vi "Create Arbitrary Waveform.vi"(4 "Arbitrary Waveform Data":dbl[](array[numeric]), 6 "Arbitrary Waveform Name (ARB1)":string="ARB1", 8 "error in (no error)":errorcluster, 9 "Timeout (10000 ms)":i32=10000, 10 "Channel (1: 1)":i32(ring)=1 items=["1"=1, "2"=2], 11 "VISA resource name":refnum<visa-resource-name>) -> (0 "error out":errorcluster, 3 "VISA resource name out":refnum<visa-resource-name>)   [LabVIEW 2017, in "Agilent 3352X Series.lvlib"]
doc: "Creates and saves an arbitrary (user-defined) waveform in volatile memory. \n\n<B>Note</B>: \n(1) You must specify at least 7 numbers for waveform data\n(2) Call Configure Arbitrary Waveform VI to activate it and change the settings.\n(3) Volatile memory will be cleared when you turn off your instrument or call Load State.vi.\n(4)You can store current loaded arb to non-volatile memory using Store Arbitrary Waveform.vi"
uses:
  Doppia_Freq_Circuito/Agilent 3352X Series/Agilent 3352X Series.lvlib
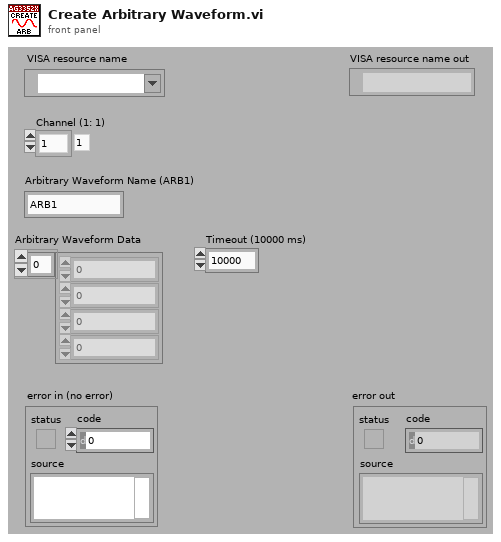
[diagram p1: front panel]
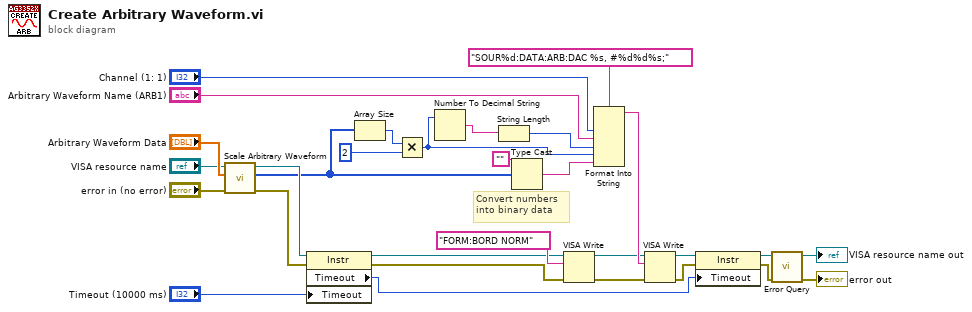
[diagram p0: block diagram]
diagram:
  # "Convert numbers\ninto binary data"
  n1 = call "Scale Arbitrary Waveform.vi"("error in (no error)"="error in (no error)", "Arbitrary Waveform Data"="Arbitrary Waveform Data", "VISA resource name"="VISA resource name") -> ("error out"=w15:errorcluster, "Scaled Arbitrary Waveform Data"=w6:i16[], "VISA resource name out"=w17:refnum<visa-resource-name>)  [unwired: 6 out]
  n2 = property class="Instr"(reference=w17, error in=w15, "Timeout"="Timeout (10000 ms)") -> (reference out=w13:refnum<visa-resource-name>, error out=w12:errorcluster, "Timeout"=w25:u32)
  n3 = Array Size(array=w6) -> (size(s)=w5:i32)
  n4 = Multiply(x=w5, y=2 ("size(s)")) -> (x*y=w3:i32)
  n5 = Number To Decimal String(number=w3) -> (decimal integer string=w2:string)  [unwired: 1 out]
  n6 = String Length(string=w2) -> (length=w1:i32)
  n7 = Type Cast(type="" ("Empty String Constant"), x=w6) -> (*(type *) &x=w7:string)
  n8 = VISA Write(VISA resource name=w13, write buffer="FORM:BORD NORM", error in (no error)=w12) -> (VISA resource name out=w11:refnum<visa-resource-name>, error out=w10:errorcluster)  [unwired: 1 out]
  n9 = Format Into String(format string="SOUR%d:DATA:ARB:DAC %s, #%d%d%s;", "Channel (1: 1)", "Arbitrary Waveform Name (ARB1)", w1, w3, w7) -> (resulting string=w27:string)  [unwired: 2 in, 1 out]
  n10 = VISA Write(VISA resource name=w11, write buffer=w27, error in (no error)=w10) -> (VISA resource name out=w22:refnum<visa-resource-name>, error out=w24:errorcluster)  [unwired: 1 out]
  n11 = property class="Instr"(reference=w22, error in=w24, "Timeout"=w25) -> (reference out=w20:refnum<visa-resource-name>, error out=w23:errorcluster)
  n12 = call "Error Query.vi"("error in (no error)"=w23, "VISA resource name"=w20) -> ("error out"=→"error out":errorcluster, "VISA resource name out"=→"VISA resource name out":refnum<visa-resource-name>)  [unwired: 8 out]
